vi "ExportFluoFit.vi"(0 "time out":dbl[](array[numeric]), 1 "lifetimes":dbl[][](array[numeric]), 2 "Lifetime Export Path (ASCII-File)":path) -> ()   [LabVIEW 2009]
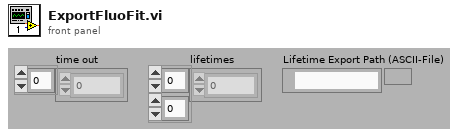
[diagram p1: front panel]
types:
  T1 = enum16{"open", "open or create", "create or replace", "create", "open (read only)"}
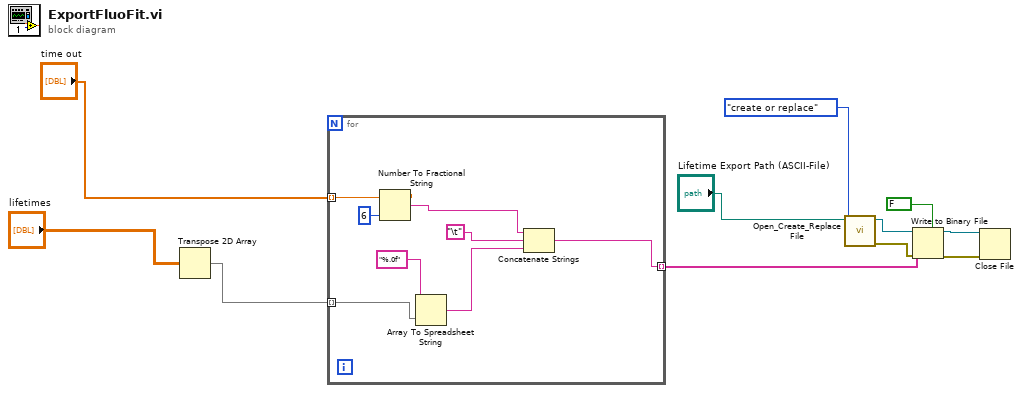
[diagram p0: block diagram]
diagram:
  n1 = Transpose 2D Array(2D array="lifetimes") -> (transposed array=w10:dbl[][])
  n2 = for {
    tunnel: w10 -> [w19] mode=indexing
    tunnel: "time out" -> [w17] mode=indexing
    tunnel: [w13] -> w2 mode=indexing
    n3 = Number To Fractional String(number=w17, precision (6)=i16 6 ("Genauigkeit (6)")) -> (F-format string=w16:string)  [unwired: 2 in]
    n4 = Array To Spreadsheet String(array=w19, 3:"%.0f" ("format (%.3f)")) -> (spreadsheet string=w15:string)  [unwired: 1 in]
    n5 = Concatenate Strings(w16, "\t", w15) -> (w13:string)
  }
  n6 = call <vilib>:"Open_Create_Replace File.vi"("function (open:0)"=T1."create or replace", "file path"="Lifetime Export Path (ASCII-File)") -> ("error out"=w3:errorcluster, "refnum"=w8:refnum<file>)  [unwired: 6 in, 2 out]
  n7 = Write to Binary File(file (use dialog)=w8, data=w2, error in=w3, 5:FALSE ("prepend array or string size? (T)")) -> (refnum out=w5:refnum<file>, error out=w4:errorcluster)  [unwired: 2 in, 1 out]
  n8 = Close File(refnum=w5, error in=w4) -> ()  [unwired: 2 out]
